vi "Spartan Config.vi"(10 "Default Value (\"\")":string, 11 "Config Key (\"\")":string) -> (2 "Found Key?":bool, 3 "Config Value":string, 5 "CONFIG":T1)   [LabVIEW 2011]
uses:
  ITK EXT/utils/keyedarr.llb/Keyed Array.ctl
  Spartan CONFIG Global.vi
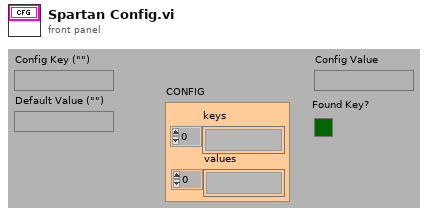
[diagram p1: front panel]
types:
  T1 = typedef "Keyed Array.ctl" = cluster{"keys":string[], "values":string[]}
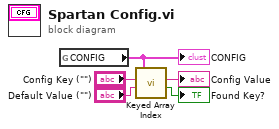
[diagram p0: block diagram]
diagram:
  n1 = global read "Spartan CONFIG Global.vi" "CONFIG"() -> (w1:T1)
  "CONFIG" <- w1
  n2 = call "Keyed Array Index.vi"("default value"="Default Value (\"\")", "key"="Config Key (\"\")", "array in"=w1) -> ("valid key"=→"Found Key?":bool, "value"=→"Config Value":string)  [unwired: 1 in, 2 out]
